vi "Analyse.vi"(8 "error in (no error)":errorcluster, 10 "ImageData":T1, 11 "FluorescenceAnalyser in":refnum<class "FluorescenceAnalyser.lvclass">) -> (0 "error out":errorcluster, 3 "FluorescenceAnalyser out":refnum<class "FluorescenceAnalyser.lvclass">)   [LabVIEW 2011, in "Tools.lvlib" / "Imaging.lvlib" / "FluorescenceAnalyser.lvclass"]
uses:
  FluorescenceAnalyser.lvclass
  FluorescenceAnalyser.lvclass/FluorescenceAnalyser.ctl
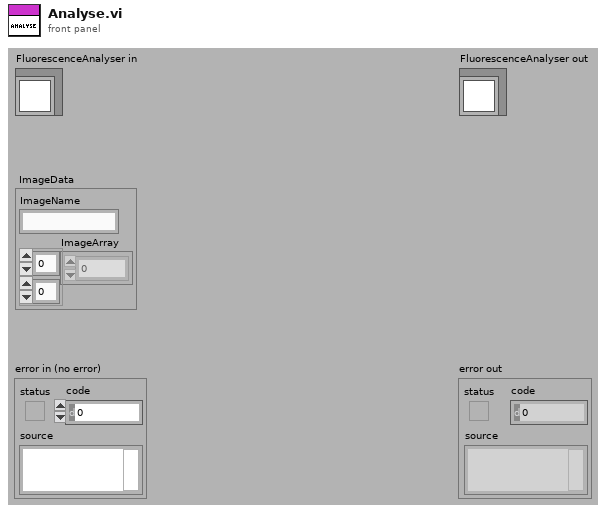
[diagram p1: front panel]
types:
  T1 = cluster{"ImageName":string, "ImageArray":sgl[][]}
  T2 = cluster{"ImageName":string, "ImageArray":sgl[][]}[]
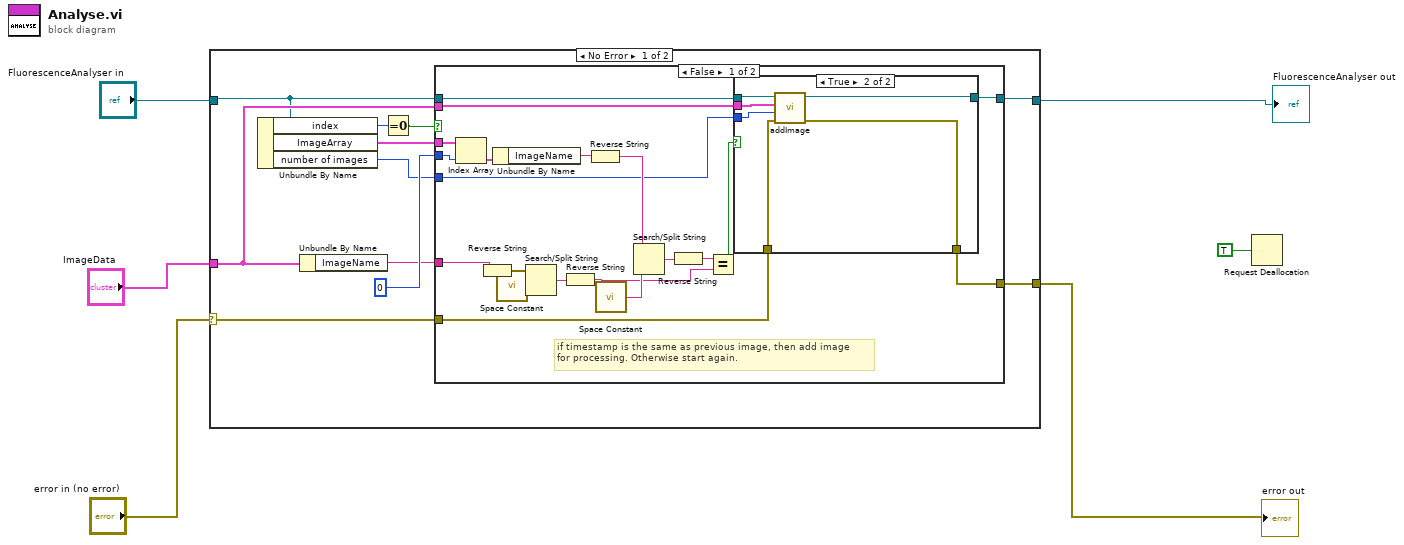
[diagram p0: block diagram]
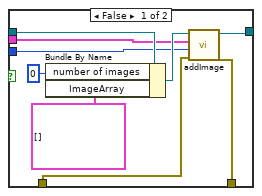
[diagram p2: hidden frame]
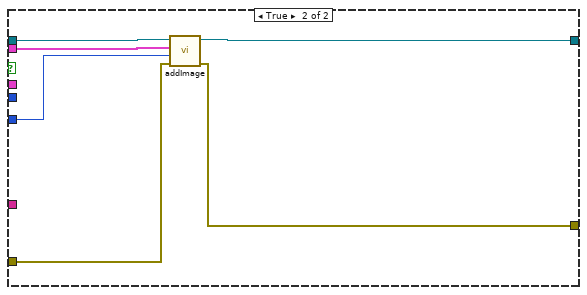
[diagram p3: hidden frame]
diagram:
  n1 = case shown="No Error" "error in (no error)" {
    selector: "error in (no error)" -> [w16 w59]
    tunnel: [w15 w59] -> w3
    tunnel: [w17 w60] -> w4
    tunnel: "FluorescenceAnalyser in" -> [w13 w60]
    tunnel: "ImageData" -> [w14 _]
    frame No Error {
      n2 = Unbundle By Name(w13) -> ("index"=w9:i32, "ImageArray"=w12:T2, "number of images"=w7:i32)
      n3 = Unbundle By Name(w14) -> ("ImageName"=w8:string)
      n4 = Equal To 0?(x=w9) -> (x = 0?=w10:bool)
      n5 = case shown="False" w10 {
        tunnel: [w22 w57] -> w17
        tunnel: w16 -> [w20 w56]
        tunnel: [w19 w55] -> w15
        tunnel: w14 -> [w21 w54]
        tunnel: w13 -> [w23 w58]
        tunnel: w12 -> [w36 _]
        tunnel: 0 -> [w37 _]
        tunnel: w8 -> [w27 _]
        tunnel: w7 -> [w18 w53]
        frame False {
          # "if timestamp is the same as previous image, then add image\nfor processing. Otherwise start again."
          n6 = Index Array(array=w36, index=w37) -> (element=w35:T1)
          n7 = Reverse String(1:w27) -> (0:w30:string)
          n8 = Unbundle By Name(w35) -> ("ImageName"=w34:string)
          n9 = call <vilib>:"Space Constant.vi"() -> ("String"=w29:string)
          n10 = Search/Split String(string=w30, search string/char (-)=w29) -> (match + rest of string=w28:string)  [unwired: 1 in, 2 out]
          n11 = Reverse String(1:w28) -> (0:w25:string)
          n12 = Reverse String(1:w34) -> (0:w33:string)
          n13 = call <vilib>:"Space Constant.vi"() -> ("String"=w32:string)
          n14 = Search/Split String(string=w33, search string/char (-)=w32) -> (match + rest of string=w31:string)  [unwired: 1 in, 2 out]
          n15 = Reverse String(1:w31) -> (0:w26:string)
          n16 = Equal?(x=w26, y=w25) -> (x = y?=w24:bool)
          n17 = case shown="True" w24 {
            tunnel: w23 -> [w45 w52]
            tunnel: [w38 w51] -> w22
            tunnel: w21 -> [w42 w50]
            tunnel: w20 -> [w40 w49]
            tunnel: [w39 w48] -> w19
            tunnel: w18 -> [w41 w47]
            frame False {
              n18 = Bundle By Name(cluster=w45, "number of images"=0, "ImageArray"=T2 []) -> (w43:refnum<class "FluorescenceAnalyser.lvclass">)
              n19 = call "addImage.vi"("error in (no error)"=w40, "number of images"=w41, "ImageData"=w42, "FluorescenceAnalyser in"=w43) -> ("error out"=w39:errorcluster, "FluorescenceAnalyser out"=w38:refnum<class "FluorescenceAnalyser.lvclass">)  [unwired: 6 in]
            }
            frame True {
              n20 = call "addImage.vi"("error in (no error)"=w49, "number of images"=w47, "ImageData"=w50, "FluorescenceAnalyser in"=w52) -> ("error out"=w48:errorcluster, "FluorescenceAnalyser out"=w51:refnum<class "FluorescenceAnalyser.lvclass">)  [unwired: 6 in]
            }
          }
        }
        frame True {
          n21 = call "addImage.vi"("error in (no error)"=w56, "number of images"=w53, "ImageData"=w54, "FluorescenceAnalyser in"=w58) -> ("error out"=w55:errorcluster, "FluorescenceAnalyser out"=w57:refnum<class "FluorescenceAnalyser.lvclass">)  [unwired: 6 in]
        }
      }
    }
    frame Error {
    }
  }
  "error out" <- w3
  "FluorescenceAnalyser out" <- w4
  n22 = Request Deallocation(TRUE ("flag")) -> ()
